vi "Flywheel_Set.vi"   [LabVIEW 2019]
uses:
  Flywheel_States.ctl
  Globals/Flywheel_Globals.vi
types:
  T1 = typedef "Flywheel_States.ctl" = enum16{"No-Op", "Percent_Voltage", "Speed_Control_Manual", "Speed_Control_Auto"}
  T2 = typedef "Flywheel_Cluster.ctl" = cluster{"Flywheel_Throttle":dbl, "Control_States":T1, "Auto_Speed":bool, "Flywheel_On":bool}
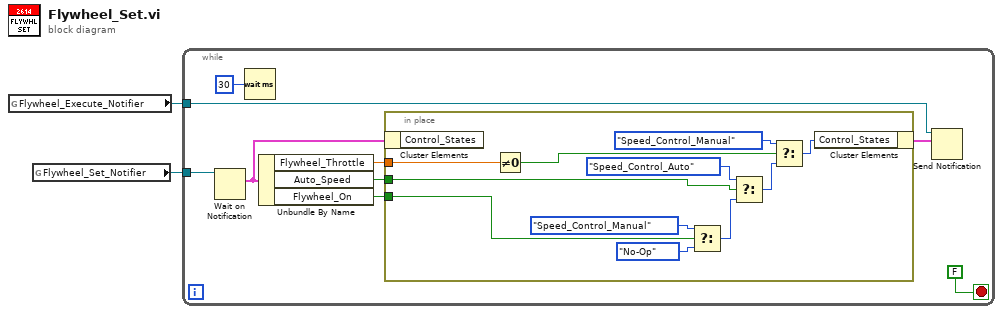
[diagram p0: block diagram]
diagram:
  n1 = global read "Flywheel_Globals.vi" "Flywheel_Execute_Notifier"() -> (w1:refnum<notifier>)
  n2 = global read "Flywheel_Globals.vi" "Flywheel_Set_Notifier"() -> (w2:refnum<notifier>)
  n3 = while {
    tunnel: w2 -> [w11]
    tunnel: w1 -> [w6]
    stop <- FALSE stop-if-true
    n4 = Wait on Notification(notifier=w11) -> (notification=w10:T2)  [unwired: 3 in, 3 out]
    n5 = Wait (ms)(milliseconds to wait=u32 30) -> ()  [unwired: 1 out]
    n6 = Unbundle By Name(w10) -> ("Flywheel_Throttle"=w9:dbl, "Auto_Speed"=w7:bool, "Flywheel_On"=w8:bool)
    n7 = in-place {
      in-place-border: w9 -> [w22]
      in-place-border: w8 -> [w21]
      in-place-border: w7 -> [w12]
      n8 = in-place-cluster #1(w10) -> ()  [unwired: 1 out]
      n9 = Not Equal To 0?(x=w22) -> (x != 0?=w15:bool)
      n10 = Select(t=Flywheel_States."Speed_Control_Manual" ("Control_States"), s=w21, f=Flywheel_States."No-Op" ("Control_States")) -> (s? t:f=w20:T1)
      n11 = Select(t=Flywheel_States."Speed_Control_Auto" ("Control_States"), s=w12, f=w20) -> (s? t:f=w16:T1)
      n12 = Select(t=Flywheel_States."Speed_Control_Manual" ("Control_States"), s=w15, f=w16) -> (s? t:f=w13:T1)
      n13 = in-place-cluster #1("Control_States"=w13) -> (w5:T2)
    }
    n14 = Send Notification(notification=w5, notifier=w6) -> ()  [unwired: 1 in, 2 out]
  }
